vi "Generate multi-line AO sequence for ref frame.vi"(6 "Cluster":T1={"Pockels ON \"Pre\" (samples)"=2, "Direction (+-Inf)"=enum."No rounding", "Additional duration to stay ON (samples)"=0, "Not the last ROI"=FALSE}, 9 "Previous excess us (us)":dbl, 11 "Variables":T3 {"Dwell time" format="%#_6f"; "Sample Clock Rate" format="%#_6f"}) -> (0 "Excess (us)":dbl, 1 "Points in o/p sequence":i32 format="%.0f points", 2 "Output sequence length (ms)":dbl format="%#_g ms", 3 "Pockels modulation sequence":dbl[](array[numeric]), 4 "Theoretical acquisition duration of ref frame (us)":dbl)   [LabVIEW 2020]
uses:
  Typedefs/Pockels mod gen variables cluster.ctl
  Typedefs/Imaging Protocols enum.ctl
  Typedefs/Pockels modulation Internal cluster 1.ctl
  Typedefs/Rounding type.ctl
  Globals/gl_Pockels control globals.vi
  Global Variables/General Globals.vi
panel:
  out "Theoretical corrected duration of ref frame AO sequence (us)":dbl
  out "Multi-line pockels modulation waveform":dbl[](graph)
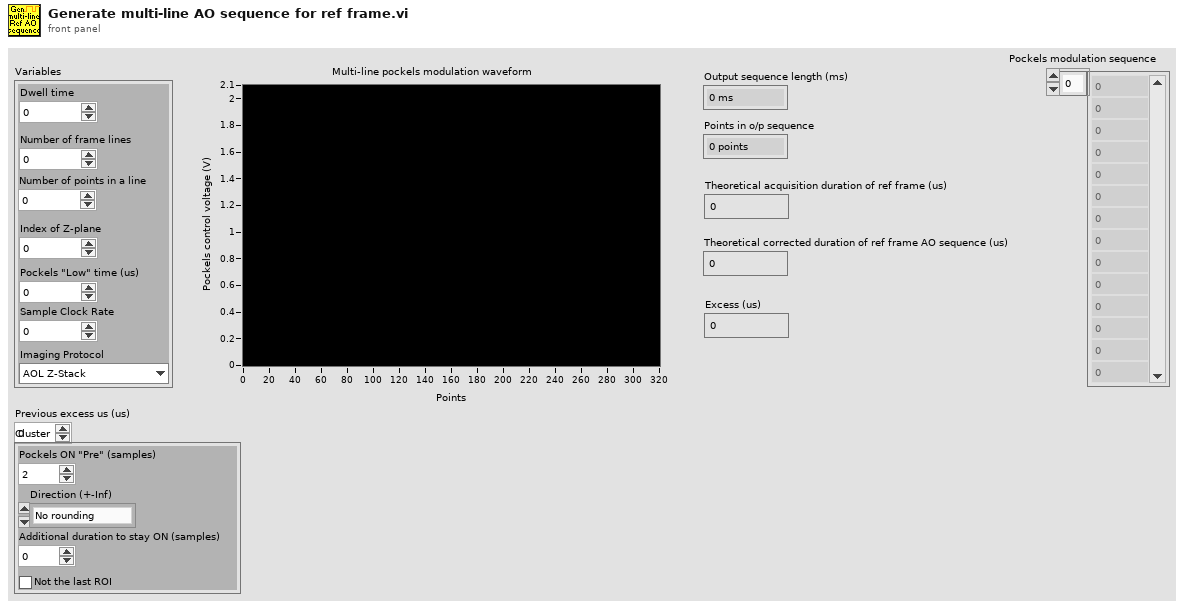
[diagram p1: front panel]
types:
  T1 = typedef "Pockels modulation Internal cluster 1.ctl" = cluster{"Pockels ON \"Pre\" (samples)":i32, "Direction (+-Inf)":T2, "Additional duration to stay ON (samples)":i32, "Not the last ROI":bool}
  T2 = typedef "Rounding type.ctl" = enum16{"No rounding", "Toward +Inf", "Toward -Inf"}
  T3 = typedef "Pockels mod gen variables cluster.ctl" = cluster{"Dwell time":dbl, "Number of frame lines":i32, "Number of points in a line":i32, "Index of Z-plane":i32, "Pockels \"Low\" time (us)":dbl, "Sample Clock Rate":dbl, "Imaging Protocol":T4}
  T4 = typedef "Imaging Protocols enum.ctl" = enum16{"AOL Z-Stack", "Motor Z Stack", "Functional Acquisition", "Single Plane Acquisition", "Volume Acquisition", "Live Imaging", "Live Plane Imaging", "Live Volume Imaging"}
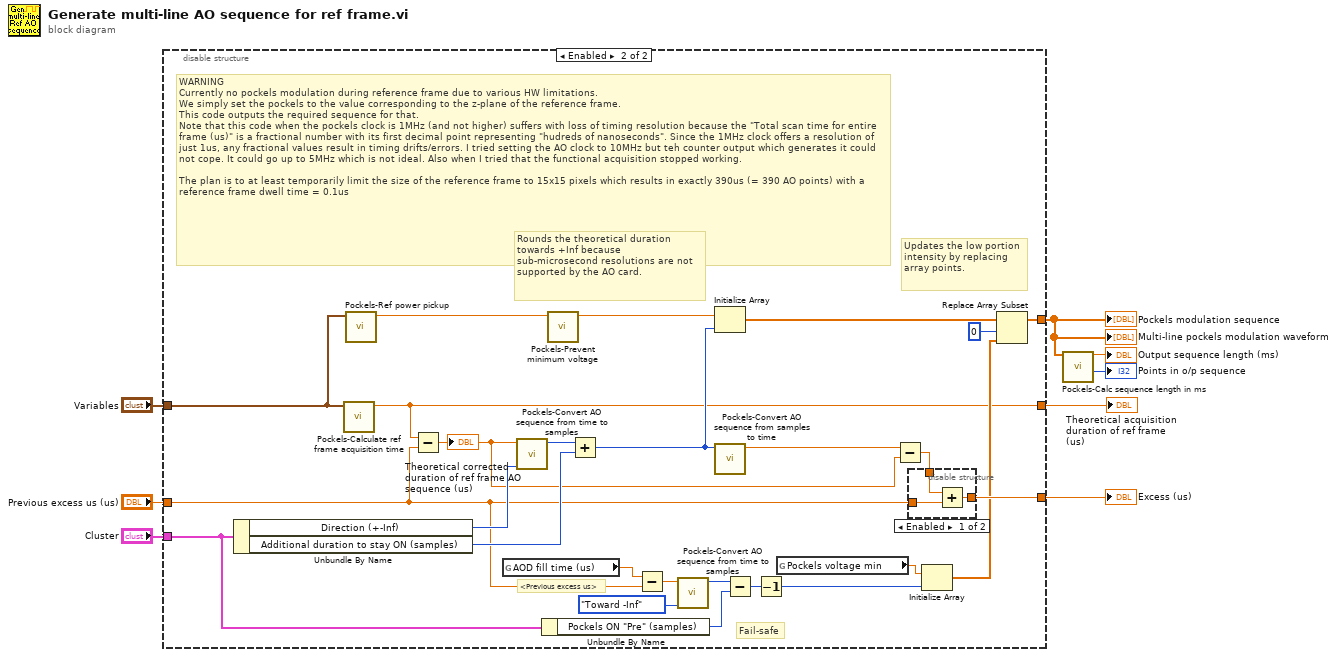
[diagram p0: block diagram]
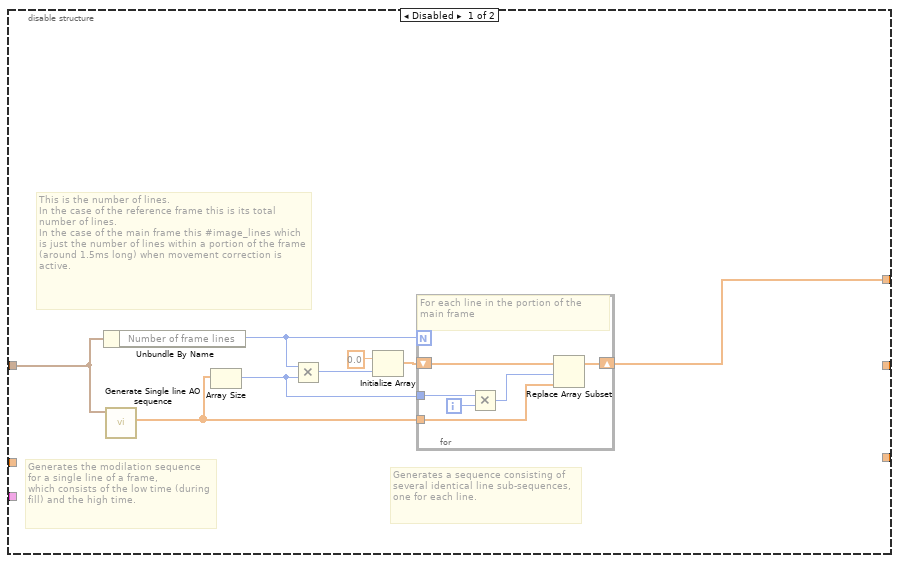
[diagram p2: hidden frame]
diagram:
  n1 = disable-structure shown="Enabled" {
    disable-tunnel: "Variables" -> [w9 w26]
    disable-tunnel: [w10 w28] -> w6
    disable-tunnel: "Previous excess us (us)" -> [_ w34]
    disable-tunnel: "Cluster" -> [_ w31]
    disable-tunnel: [_ w41] -> w2
    disable-tunnel: [_ w25] -> w1
    frame Disabled {
      # "This is the number of lines.\nIn the case of the reference frame this is its total number of lines.\nIn the case of the main frame this #image_lines which is just the number of lines within a portion of the frame (around 1.5ms long) when movement correction is active."
      # "Generates a sequence consisting of several identical line sub-sequences, one for each line."
      # "Generates the modilation sequence for a single line of a frame,\nwhich consists of the low time (during fill) and the high time."
      n2 = Unbundle By Name(w9) -> ("Number of frame lines"=w11:i32)
      n3 = call "Generate Single line AO sequence.vi"("Variables"=w9) -> ("Single line AO sequence"=w15:dbl[])  [unwired: 10 in]
      n4 = Array Size(array=w15) -> (size(s)=w16:i32)
      n5 = Multiply(x=w11, y=w16) -> (x*y=w12:i32)
      n6 = Initialize Array(0.0 ("Pockels Value (minimum prevented)"), w12) -> (w14:dbl[])
      n7 = for {
        N: w11 -> [_]
        tunnel: w15 -> [w17]
        shift-right: [w21] -> w10
        shift-left: w14 -> [w22]
        tunnel: w16 -> [w19]
        i -> [w20]
        # "For each line in the portion of the main frame"
        n8 = Multiply(x=w19, y=w20) -> (x*y=w18:i32)
        n9 = Replace Array Subset(array=w22, new element=w17, index=w18) -> (w21:dbl[])
      }
    }
    frame Enabled {
      # "Updates the low portion intensity by replacing array points."
      # "<Previous excess us>"
      # "Rounds the theoretical duration towards +Inf because sub-microsecond resolutions are not supported by the AO card."
      # "Fail-safe"
      # "WARNING\nCurrently no pockels modulation during reference frame due to various HW limitations.\nWe simply set the pockels to the value corresponding to the z-plane of the reference frame.\nThis code outputs the required sequence for that.\nNote that this code when the pockels clock is 1MHz (and not higher) suffers with loss of timing resolution because the \"Total scan time for entire frame (us)\" is a fractional number with its first decimal point representing \"hudreds of nanoseconds\". Since the 1MHz clock offers a resolution of just 1us, any fractional values result in timing drifts/errors. I tried setting the AO clock to 10MHz but teh counter output which generates it could not cope. It could go up to 5MHz which is not ideal. Also when I tried that the functional acquisition stopped working.\n\nThe plan is to at least temporarily limit the size of the reference frame to 15x15 pixels which results in exactly 390us (= 390 AO points) with a reference frame dwell time = 0.1us"
      n10 = Unbundle By Name(w31) -> ("Direction (+-Inf)"=w45:T2, "Additional duration to stay ON (samples)"=w44:i32)
      n11 = call "Pockels-Calculate ref frame acquisition time.vi"("Variables"=w26) -> ("Theoretical acquisition duration of ref frame (us)"=w25:dbl)  [unwired: 10 in]
      n12 = call "Pockels-Ref power pickup.vi"("Variables"=w26) -> ("Pockels high duration voltage"=w48:dbl)  [unwired: 9 in, 1 out]
      n13 = Subtract(x=w25, y=w34) -> (x-y=w23:dbl)
      "Theoretical corrected duration of ref frame AO sequence (us)" <- w23
      n14 = global read "General Globals.vi" "AOD fill time (us)"() -> (w33:dbl)
      n15 = call "Pockels-Convert AO sequence from time to samples.vi"("Direction (+Inf)"=w45, "Duration of AO sequence (us)"=w23) -> ("Number of samples in AO sequence"=w46:i32)  [unwired: 9 in]
      n16 = Unbundle By Name(w31) -> ("Pockels ON \"Pre\" (samples)"=w32:i32)
      n17 = call "Pockels-Prevent minimum voltage.vi"("Pockels Value"=w48) -> ("Pockels Value (minimum prevented)"=w47:dbl)  [unwired: 8 in, 2 out]
      n18 = Add(x=w46, y=w44) -> (x+y=w43:i32)
      n19 = Subtract(x=w33, y=w34) -> (x-y=w38:dbl)
      n20 = call "Pockels-Convert AO sequence from time to samples.vi"("Direction (+Inf)"=Rounding_type."Toward -Inf", "Duration of AO sequence (us)"=w38) -> ("Number of samples in AO sequence"=w35:i32)  [unwired: 9 in]
      n21 = Initialize Array(w47, w43) -> (w29:dbl[])
      n22 = call "Pockels-Convert AO sequence from samples to time.vi"("Number of samples in AO sequence"=w43) -> ("Duration of AO sequence (us)"=w24:dbl)  [unwired: 10 in]
      n23 = Subtract(x=w35, y=w32) -> (x-y=w36:i32)
      n24 = Decrement(x=w36) -> (x-1=w37:i32)
      n25 = global read "gl_Pockels control globals.vi" "Pockels voltage min"() -> (w39:dbl)
      n26 = Subtract(x=w24, y=w23) -> (x-y=w42:dbl)
      n27 = disable-structure shown="Enabled" {
        disable-tunnel: w42 -> [w51 w52]
        disable-tunnel: [w50 w52] -> w41
        disable-tunnel: w34 -> [w49 _]
        frame Enabled {
          n28 = Add(x=w51, y=w49) -> (x+y=w50:dbl)
        }
        frame Disabled {
        }
      }
      n29 = Initialize Array(w39, w37) -> (w27:dbl[])
      n30 = Replace Array Subset(array=w29, new element=w27, index=0) -> (w28:dbl[])
    }
  }
  "Pockels modulation sequence" <- w6
  "Multi-line pockels modulation waveform" <- w6
  "Excess (us)" <- w2
  "Theoretical acquisition duration of ref frame (us)" <- w1
  n31 = call "Pockels-Calc sequence length in ms.vi"("Pockels modulation sequence in"=w6) -> ("Sequence length (points)"=→"Points in o/p sequence":i32, "Sequence length (ms)"=→"Output sequence length (ms)":dbl)  [unwired: 8 in, 1 out]
